vi "Send Message.vi"(6 "ID":string, 8 "error in (no error)":errorcluster, 9 "Data":variant, 10 "Command":string, 11 "RemoteControl.STM in":refnum<class "RemoteControl.STM.lvclass">) -> (0 "error out":errorcluster, 3 "RemoteControl.STM out":refnum<class "RemoteControl.STM.lvclass">)   [LabVIEW 2019, in "RemoteControl.STM.lvclass"]
uses:
  RemoteControl.STM.lvclass
  C:/Program Files (x86)/National Instruments/LabVIEW 2019/user.lib/LevyLab/RemoteControl/RemoteControl/RemoteControl.lvclass
  <vilib>/NI/STM/TCP/TCP Write Options.ctl
  <userlib>/LevyLab/RemoteControl/RemoteControl/RemoteControl.lvclass/RemoteControl.ctl
  RemoteControl.STM.lvclass/RemoteControl.STM.ctl
  <vilib>/NI/STM/TCP/Get Connection Reference (TCP).vi
  <vilib>/NI/STM/TCP/Write Message (TCP).vi
  <vilib>/NI/STM/Connection Manager/TCP/TCP Connection Manager.vi
  <vilib>/NI/STM/NI STM.lvlib
  <userlib>/LevyLab/RemoteControl/RemoteControl/RemoteControl.lvclass
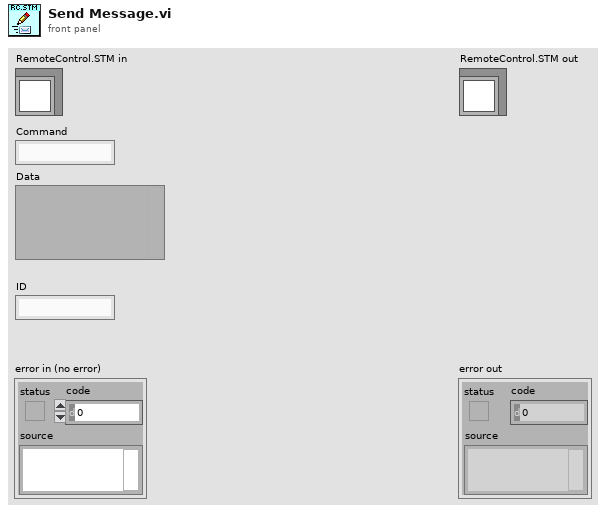
[diagram p1: front panel]
types:
  T1 = typedef "NI STM.lvlib/TCP Write Options.ctl" = cluster{"ignore timeout error":bool, "timeout ms (1000)":i32}
  T2 = typedef "NI STM.lvlib/TCP Connection Info.ctl" = cluster{"connection ID":refnum<k5>, "meta data":T3[]}
  T3 = typedef "NI STM.lvlib/MetaDataElement.ctl" = string
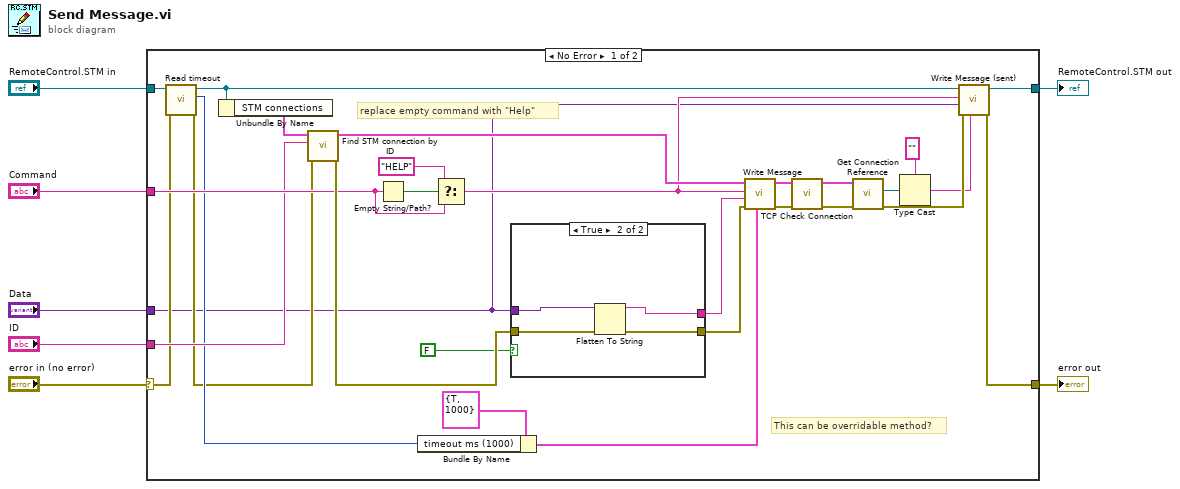
[diagram p0: block diagram]
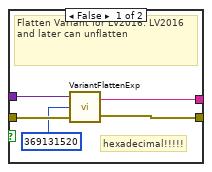
[diagram p2: hidden frame]
diagram:
  n1 = case shown="No Error" "error in (no error)" {
    selector: "error in (no error)" -> [w11 w47]
    tunnel: [w17 w47] -> w7
    tunnel: "ID" -> [w15 _]
    tunnel: "Data" -> [w8 _]
    tunnel: "Command" -> [w25 _]
    tunnel: "RemoteControl.STM in" -> [w14 w46]
    tunnel: [w21 w46] -> w2
    frame No Error {
      # "This can be overridable method?"
      # "replace empty command with \"Help\""
      n2 = call <userlib>:"Read timeout.vi"("error in (no error)"=w11, "RemoteControl in"=w14) -> ("error out"=w10:errorcluster, "timeout"=w12:i32, "RemoteControl out"=w13:refnum<class "RemoteControl.STM.lvclass">)  [unwired: 7 in]
      n3 = Unbundle By Name(w13) -> ("STM connections"=w28:T2[])
      n4 = call "Find STM connection by ID.vi"("error in"=w10, "ID"=w15, "STM connections"=w28) -> ("error out"=w31:errorcluster, "Connection Ref"=w32:T2)  [unwired: 7 in]
      n5 = Empty String/Path?(string/path=w25) -> (empty?=w34:bool)
      n6 = Bundle By Name(cluster=T1 {"ignore timeout error"=TRUE, "timeout ms (1000)"=1000} ("options"), "timeout ms (1000)"=w12) -> (w35:T1)
      n7 = Select(t="HELP", s=w34, f=w25) -> (s? t:f=w20:string)
      n8 = case shown="True" FALSE {
        tunnel: [w40 w45] -> w26
        tunnel: [w39 w44] -> w9
        tunnel: w31 -> [w41 w43]
        tunnel: w8 -> [w38 w42]
        frame False {
          # "hexadecimal!!!!!"
          # "Flatten Variant for LV2016: LV2016 and later can unflatten"
          n9 = call <vilib>:"VariantFlattenExp.vi"("error in (no error)"=w41, "version"=u32 369131520, "variant"=w38) -> ("error out"=w40:errorcluster, "data string"=w39:string)
        }
        frame True {
          n10 = Flatten To String(anything=w42, error in (no error)=w43) -> (data string=w44:string, error out=w45:errorcluster)  [unwired: 2 in, 1 out]
        }
      }
      n11 = call-poly <vilib>:"Write Message.vi"("options"=w35, "error in"=w26, "data"=w9, "name"=w20, "connection info in"=w32) -> ("error out"=w29:errorcluster, "connection info out"=w30:T2)  [unwired: 5 in]
      n12 = call <vilib>:"TCP Check Connection.vi"("error in"=w29, "connection in"=w30) -> ("error out"=w22:errorcluster, "connection out"=w24:T2)  [unwired: 7 in, 1 out]
      n13 = call-poly <vilib>:"Get Connection Reference.vi"("error in"=w22, "connection info in"=w24) -> ("error out"=w18:errorcluster, "connection ID out"=w23:refnum<k5>)  [unwired: 7 in, 1 out]
      n14 = Type Cast(type="", x=w23) -> (*(type *) &x=w16:string)
      n15 = call <userlib>:"Write Message (sent).vi"("ID (sent)"=w16, "error in (no error)"=w18, "Data"=w8, "Command (sent)"=w20, "RemoteControl in"=w13) -> ("error out"=w17:errorcluster, "RemoteControl out"=w21:refnum<class "RemoteControl.STM.lvclass">)  [unwired: 5 in]
    }
    frame Error {
    }
  }
  "error out" <- w7
  "RemoteControl.STM out" <- w2
